vi "Serial Read.vi"(8 "error in (no error)":errorcluster, 9 "Count (256)":u32=256, 10 "Node In":string, 11 "VISA resource name":refnum<visa-resource-name>) -> (0 "error out":errorcluster, 1 "Data":string, 2 "Node Out":string, 3 "VISA resource name out":refnum<visa-resource-name>, 4 "Command String":string)   [LabVIEW 2009, in "Keithley 2600 Series.lvlib"]
doc: "This VI reads data from the instrument's RS-232 serial port.\n\nThis function will read available characters from the serial port. It will not wait for new characters to arrive. As long as maxchars is a relatively small number (less than several hundred characters), all characters received by the serial port prior to the call will be returned. This might be less than maxchars. If too many characters are received in between calls to this function, the RS-232 buffers will overflow and some characters may be lost.\n\nThis function can be called as many times as necessary to receive the required num­ber of characters. For optimal performance, it is suggested that a small delay be used between repeat calls to this function.\n\nThe data returned is the raw data stream read from the port. Control characters, ter­minator characters, etc. will not be processed nor will the data stream be altered in any way.\n\nThis function cannot be used if the serial port is enabled as a command interface. A settings conflict error will be generated if the serial port is enabled as a command interface when this function is called.\n\n<b>Functions and Attributes Used</b>\nserial.read()"
uses:
  <instrlib>/Keithley 2600 Series/Keithley 2600 Series.lvlib
  <instrlib>/Keithley 2600 Series/Private/GlobalVariables.vi
panel:
  # "(c) 2008 Keithley Instruments, Inc.  ALL RIGHTS RESERVED."
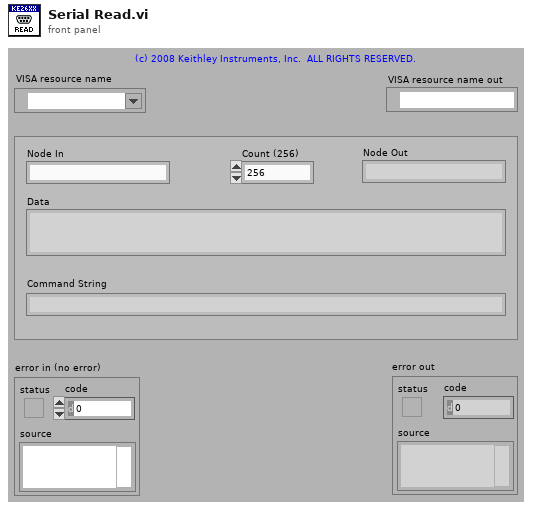
[diagram p1: front panel]
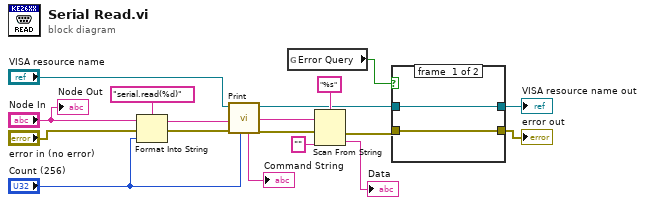
[diagram p0: block diagram]
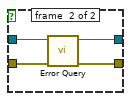
[diagram p2: hidden frame]
diagram:
  n1 = Format Into String(format string="serial.read(%d)", initial string="Node In", error in="error in (no error)", "Count (256)") -> (resulting string=w8:string, error out=w7:errorcluster)
  n2 = call <instrlib>:"Print.vi"("Byte Count (1024)"="Count (256)", "error in (no error)"=w7, "Input"=w8, "VISA resource name"="VISA resource name") -> ("error out"=w2:errorcluster, "Output"=w3:string, "VISA resource name out"=w1:refnum<visa-resource-name>, "Command String"=→"Command String":string)  [unwired: 1 in, 3 out]
  n3 = global read "GlobalVariables.vi" "Error Query"() -> (w15:bool)
  n4 = Scan From String(format string="%s", input string=w3, error in=w2, default 1="" ("default value 1")) -> (error out=w14:errorcluster, output 1=→"Data":string)  [unwired: 1 in, 2 out]
  n5 = case shown="True" w15 {
    tunnel: w14 -> [w20 w24]
    tunnel: [w19 w22] -> w13
    tunnel: [w20 w23] -> w12
    tunnel: w1 -> [w19 w21]
    frame #0 {
    }
    frame #1 {
      n6 = call <instrlib>:"Error Query.vi"("error in (no error)"=w24, "VISA resource name"=w21) -> ("error out"=w23:errorcluster, "VISA resource name out"=w22:refnum<visa-resource-name>)  [unwired: 1 in, 7 out]
    }
  }
  "VISA resource name out" <- w13
  "error out" <- w12
  "Node Out" <- "Node In"
